vi "computer_GUI.vi"(11 "GUI_cluster":T2={"Sub Panel"=refnum, "GUIdevice"="Bella_LP_Mode", "CtlRef"=refnum, "User Event in"=refnum}) -> ()   [LabVIEW 2013]
uses:
  Shared/GUI_Template/GUI_master/tcp new data cluster.ctl
  Controls/eventtypdef1.ctl
  <vilib>/Utility/miscctls.llb/LVRangeTypeDef.ctl
  Shared/GUI_Template/GUI_master/tcp_new_data_event.ctl
  Controls/GUI_cluster.ctl
panel:
  out "Slide 2":u8(slide) scale=0.0..100.0
  in  "Refresh Button":bool
  in  "check coputers":bool=TRUE
  out "All on?":bool
  out "Computers not on":string[](array[string])
  out "off computers":string[](array[string])
  in  "Ping type":T1(ring)
  in  "IP Addresses":string[](array[string])
  in  "error out":errorcluster
  out "error out 2":errorcluster
  out "tcp data event":T3
  out "GUIdevice 1":string="Bella_LP_Mode"
  in  "stop":bool
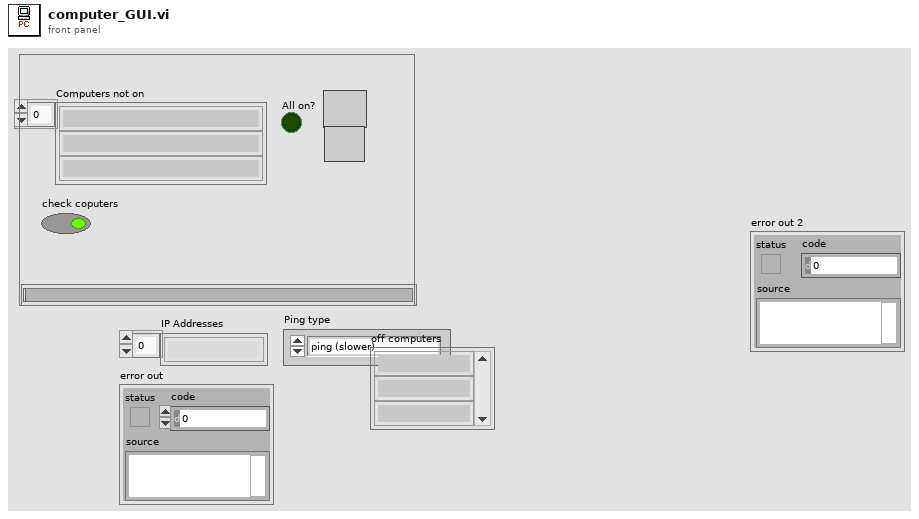
[diagram p1: front panel]
types:
  T1 = enum16{"ping (slower)", "nmap (only if installed)"}
  T2 = typedef "GUI_cluster.ctl" = cluster{"Sub Panel":refnum<vi>, "GUIdevice":string, "CtlRef":refnum<vi>, "User Event in":refnum<user-event>}
  T3 = typedef "tcp_new_data_event.ctl" = refnum<user-event>
  T4 = typedef "eventtypdef1.ctl" = cluster{"label":string, "Sub Panel":refnum<vi>, "CtlRef":refnum<vi>, "This VI":refnum<vi>}
  T5 = typedef "tcp new data cluster.ctl" = cluster{"EventEnum":enum16{"new data", "connection status update"}, "Device name":string}
  T6 = typedef "LVRangeTypeDef.ctl" = cluster{"Minimum":dbl, "Maximum":dbl, "Increment":dbl, "Minor Increment":dbl, "Start":dbl}
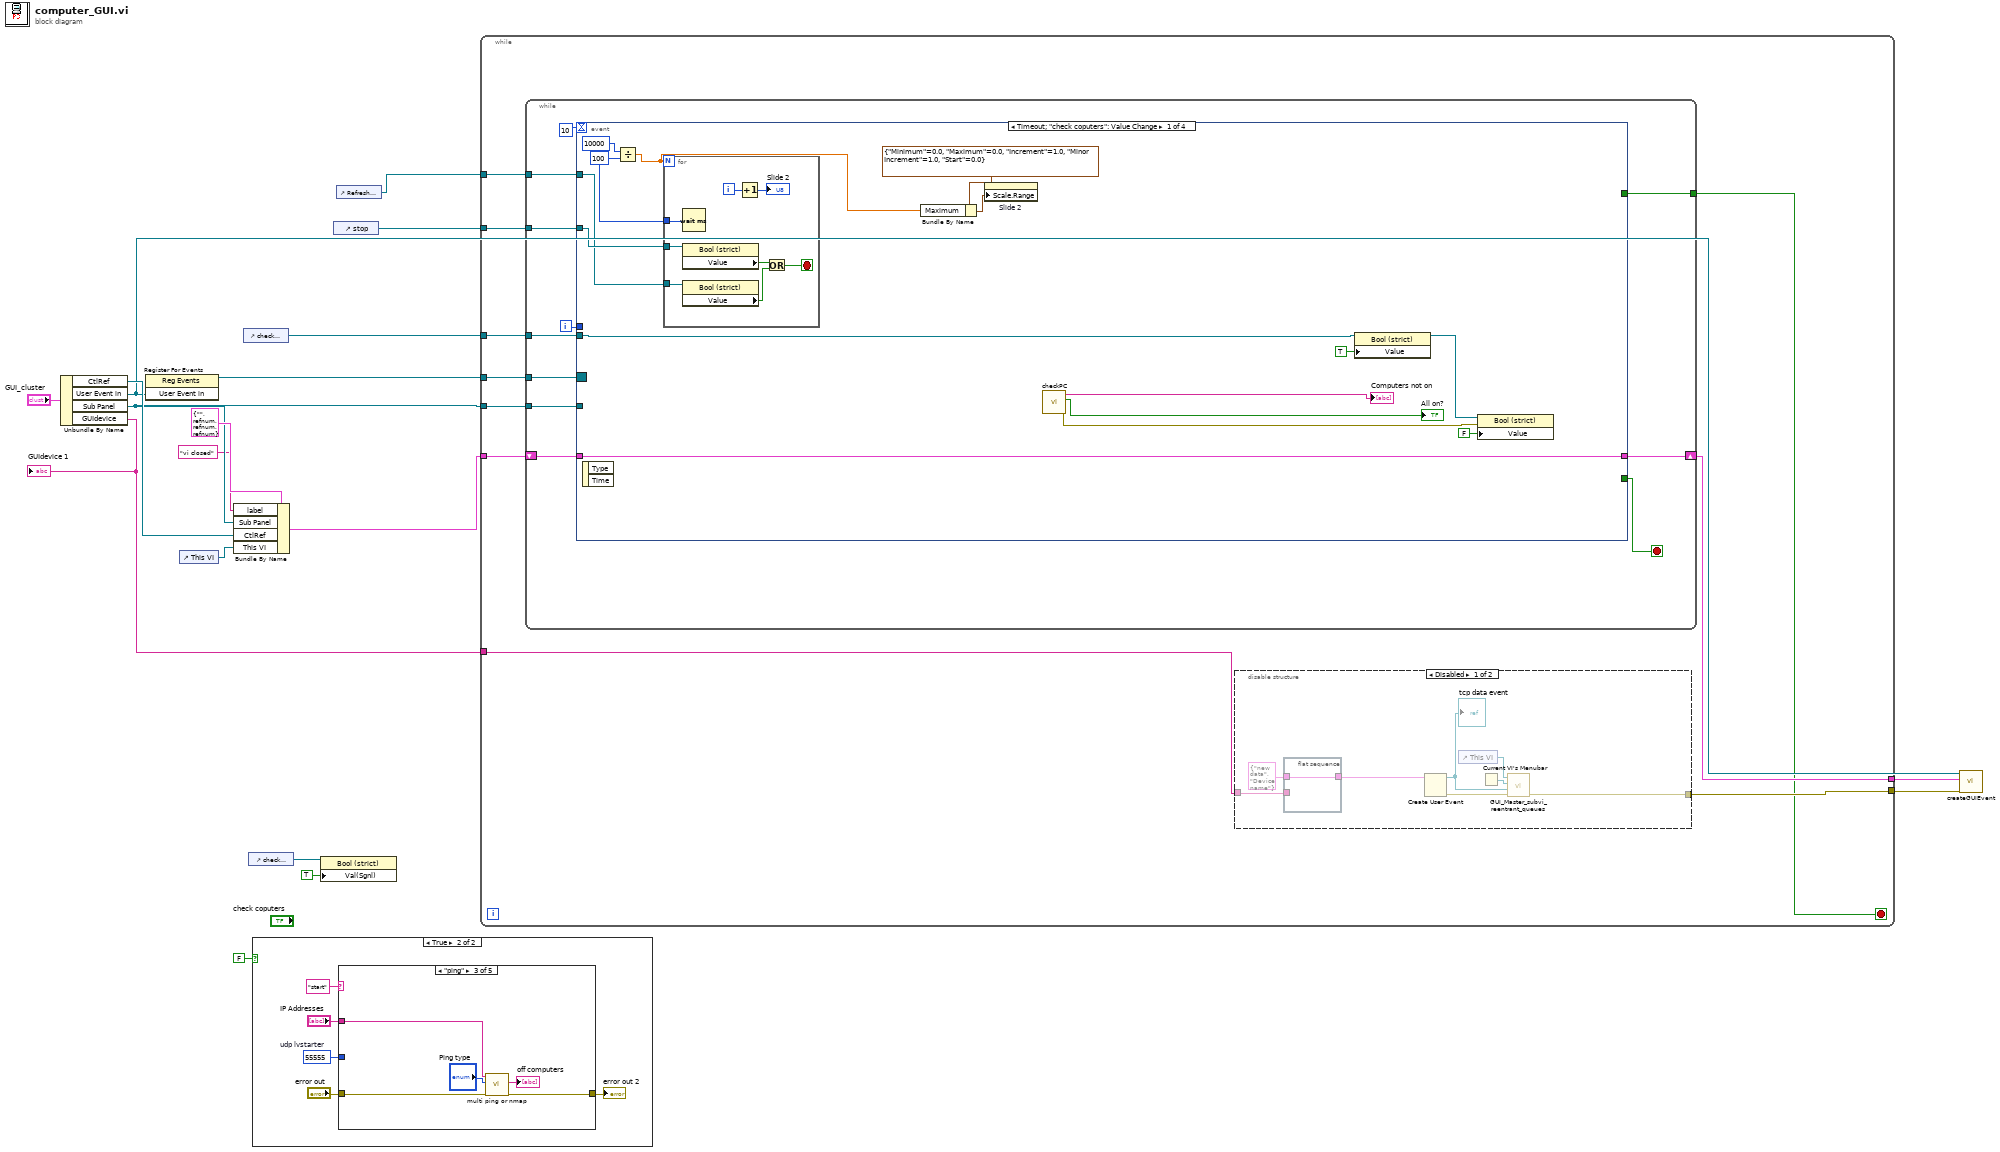
[diagram p0: block diagram]
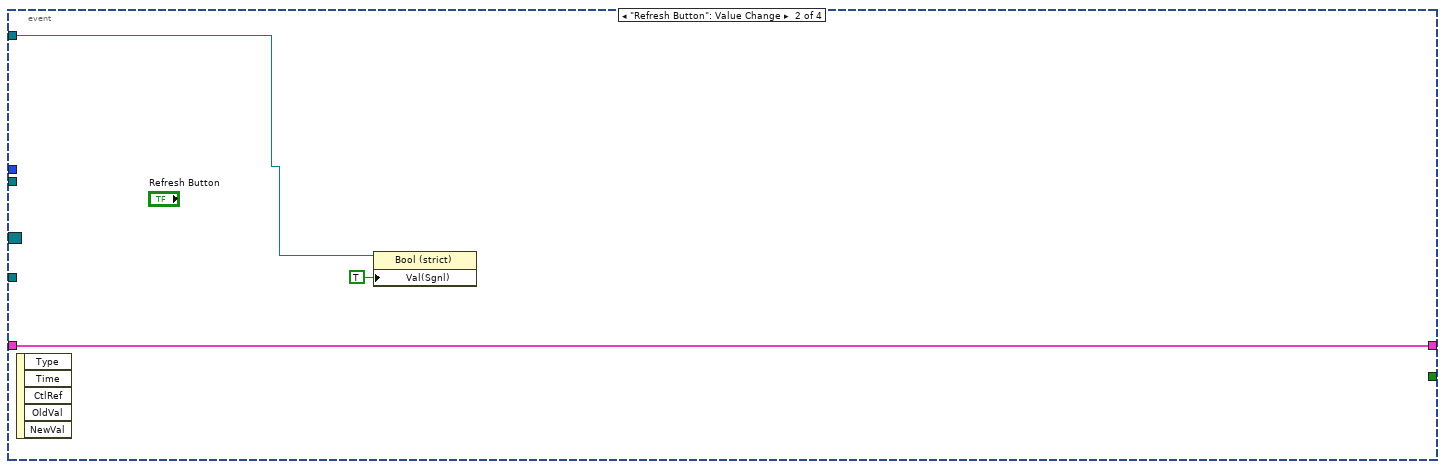
[diagram p3: hidden frame]
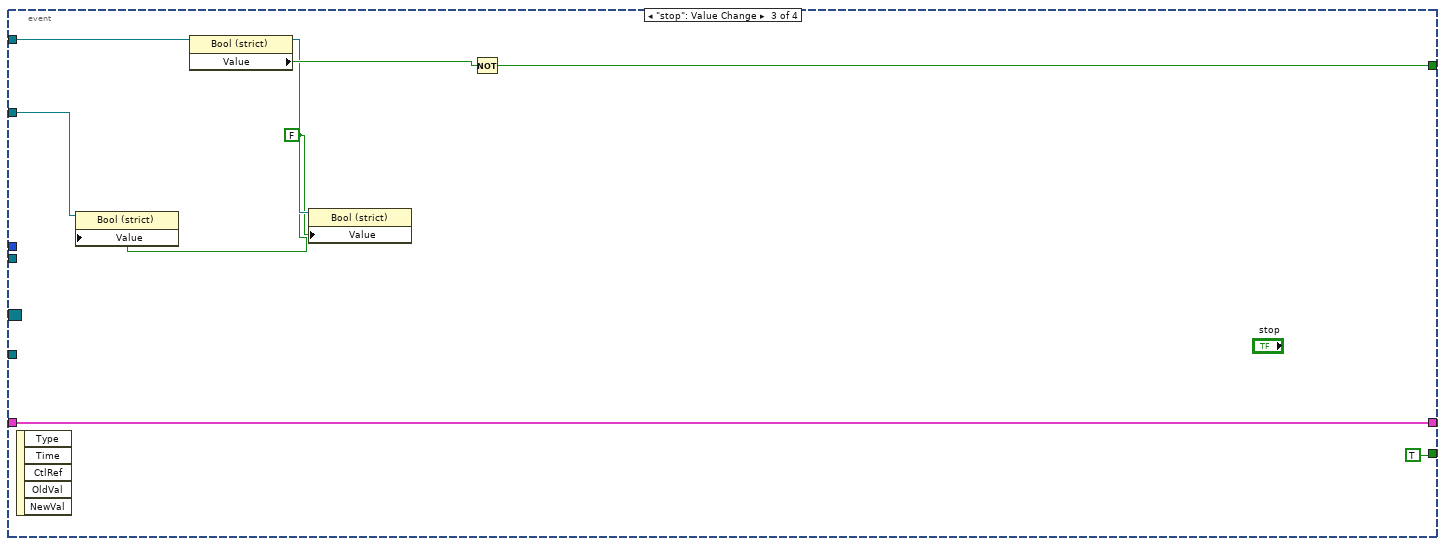
[diagram p4: hidden frame]
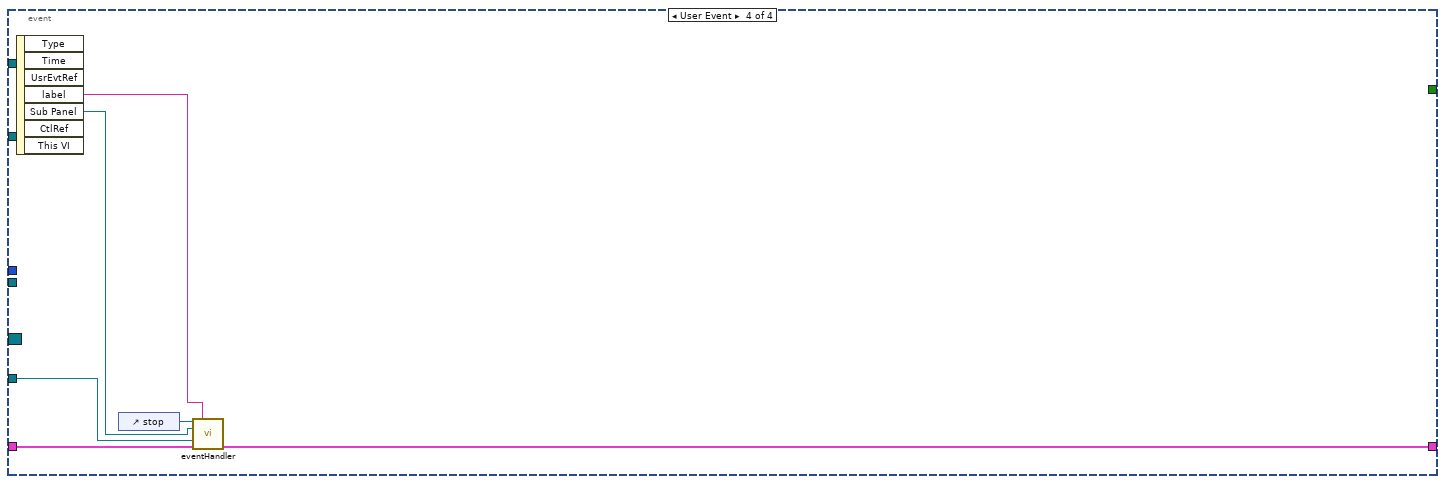
[diagram p5: hidden frame]
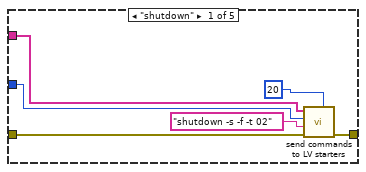
[diagram p7: hidden frame]
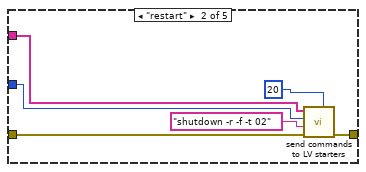
[diagram p8: hidden frame]
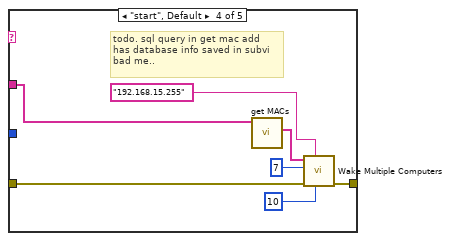
[diagram p9: hidden frame]
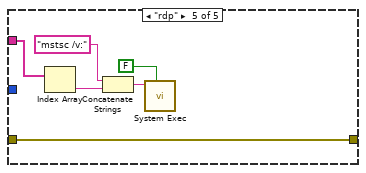
[diagram p10: hidden frame]
diagram:
  n1 = Unbundle By Name("GUI_cluster") -> ("CtlRef"=w16:refnum<vi>, "User Event in"=w11:refnum<user-event>, "Sub Panel"=w9:refnum<vi>, "GUIdevice"=w14:string)
  "GUIdevice 1" <- w14
  n2 = register-events(w11) -> (reference out=w10:refnum<event-registration>)  [unwired: 2 in, 1 out]
  n3 = control-ref of="This VI"() -> (w15:refnum<vi>)
  n4 = Bundle By Name(cluster=T4 {"label"="", "Sub Panel"=refnum, "CtlRef"=refnum, "This VI"=refnum} ("event data"), "label"="vi closed", "Sub Panel"=w9, "CtlRef"=w16, "This VI"=w15) -> (w12:T4)
  n5 = control-ref of="check coputers"() -> (w3:refnum<vi>)
  n6 = control-ref of="check coputers"() -> (w5:refnum<vi>)
  n7 = case shown="True" FALSE {
    frame False {
    }
    frame True {
      w20 = u16 55555  # udp lvstarter
      n8 = case shown="\"ping\"" "start" {
        tunnel: "IP Addresses" -> [w29 w35 w39 w43 w51]
        tunnel: w20 -> [w28 w34 _ _ _]
        tunnel: "error out" -> [w26 w32 w36 w45 w53]
        tunnel: [w25 w31 w38 w44 w53] -> w21
        frame "shutdown" {
          n9 = call "send commands to LV starters.vi"("IP Addresses"=w29, "Local Port"=w28, "Message"="shutdown -s -f -t 02", "error in"=w26, "time between commands (ms)"=u32 20) -> ("error out"=w25:errorcluster)  [unwired: 3 in, 1 out]
        }
        frame "restart" {
          n10 = call "send commands to LV starters.vi"("IP Addresses"=w35, "Local Port"=w34, "Message"="shutdown -r -f -t 02", "error in"=w32, "time between commands (ms)"=u32 20) -> ("error out"=w31:errorcluster)  [unwired: 3 in, 1 out]
        }
        frame "ping" {
          n11 = call "multi ping or nmap.vi"("error in (no error)"=w36, "Ping type"="Ping type", "IP Addresses"=w39) -> ("error out"=w38:errorcluster, "Computers not on"=→"off computers":string[])  [unwired: 2 in, 1 out]
        }
        frame "start", Default {
          # "todo. sql query in get mac add\nhas database info saved in subvi\nbad me.."
          n12 = call "get MACs.vi"("IP Addresses to..."=w43) -> ("MACs Hex"=w42:string[])  [unwired: 9 in, 1 out]
          n13 = call "Wake Multiple Computers.vi"("wait in between [ms]"=u32 10, "Broadcast IP-address"="192.168.15.255", "error in"=w45, "local port"=u16 7, "MAC Addresses to Start"=w42) -> ("error out"=w44:errorcluster)  [unwired: 6 in]
        }
        frame "rdp" {
          n14 = Index Array(array=w51) -> (element=w50:string)  [unwired: 1 in]
          n15 = Concatenate Strings("mstsc /v:" ("IP"), w50) -> (w48:string)
          n16 = call <vilib>:"System Exec.vi"("wait until completion? (T)"=FALSE, "command line"=w48) -> ()  [unwired: 4 in, 6 out]
        }
      }
      "error out 2" <- w21
    }
  }
  n17 = property class="Bool (strict)"(reference=w5, "Val(Sgnl)"=TRUE ("Value (Signaling)")) -> ()  [unwired: 1 in, 2 out]
  n18 = control-ref of="stop"() -> (w2:refnum<vi>)
  n19 = control-ref of="Refresh Button"() -> (w1:refnum<vi>)
  n20 = while {
    tunnel: w14 -> [w63]
    tunnel: [w62] -> w13
    tunnel: w12 -> [w61]
    tunnel: w10 -> [w60]
    tunnel: w9 -> [w59]
    tunnel: [w58] -> w8
    tunnel: w3 -> [w57]
    tunnel: w2 -> [w56]
    tunnel: w1 -> [w55]
    stop <- w54 stop-if-true
    n21 = while {
      shift-right: [w82] -> w58
      shift-left: w61 -> [w83]
      tunnel: w60 -> [w81]
      tunnel: w59 -> [w80]
      tunnel: w57 -> [w77]
      tunnel: w56 -> [w75]
      tunnel: w55 -> [w74]
      tunnel: [w73] -> w54
      i -> [w78]
      stop <- w76 stop-if-true
      n22 = event shown="[0] Timeout;  \"check coputers\": Value Change" {
        selector: w81 -> [_ _ _ _]
        dyn-events: _ -> [_ _ _ _]
        timeout: 10 -> [_ _ _ _]
        tunnel: [_ _ TRUE ("stop") _] -> w76
        tunnel: w83 -> [w98 w107 w117 w120]
        tunnel: [w98 w107 w117 w119] -> w82
        tunnel: w80 -> [_ _ _ w121]
        tunnel: w78 -> [_ _ _ _]
        tunnel: w77 -> [w95 _ _ _]
        tunnel: w75 -> [w85 w108 w111 _]
        tunnel: w74 -> [w84 _ w116 _]
        tunnel: [_ _ w114 _] -> w73
        event Timeout; "check coputers": Value Change {
          w87 = 100 ("y")
          n23 = event-data() -> ()  [unwired: 1 in, 2 out]
          n24 = Divide(x=10000 ("y"), y=w87) -> (x/y=w90:dbl)
          n25 = for {
            N: w90 -> [_]
            tunnel: w87 -> [w104]
            tunnel: w85 -> [w103]
            tunnel: w84 -> [w102]
            i -> [w106]
            stop <- w99 stop-if-true
            n26 = Wait (ms)(milliseconds to wait=w104) -> ()  [unwired: 1 out]
            n27 = property class="Bool (strict)"(reference=w103) -> ("Value"=w101:bool)  [unwired: 1 in, 2 out]
            n28 = property class="Bool (strict)"(reference=w102) -> ("Value"=w100:bool)  [unwired: 1 in, 2 out]
            n29 = Increment(x=w106) -> (x+1=→"Slide 2":i32)
            n30 = Or(x=w101, y=w100) -> (x .or. y?=w99:bool)
          }
          n31 = Bundle By Name(cluster=T6 {"Minimum"=0.0, "Maximum"=0.0, "Increment"=1.0, "Minor Increment"=1.0, "Start"=0.0} ("Scale.Range"), "Maximum"=w90) -> (w88:T6)
          n32 = property on="Slide 2" class="Slide (strict)"("Scale.Range"=w88) -> ()  [unwired: 2 in, 2 out]
          n33 = call "checkPC.vi"() -> ("error out"=w93:errorcluster, "All on?"=→"All on?":bool, "Computers not on"=→"Computers not on":string[])  [unwired: 9 in]
          n34 = property class="Bool (strict)"(reference=w95, "Value"=TRUE ("Value (Signaling)")) -> (reference out=w91:refnum<vi>)  [unwired: 1 in, 1 out]
          n35 = property class="Bool (strict)"(reference=w91, error in=w93, "Value"=FALSE) -> ()  [unwired: 2 out]
        }
        event "Refresh Button": Value Change {
          n36 = event-data() -> ()  [unwired: 1 in, 5 out]
          n37 = property class="Bool (strict)"(reference=w108, "Val(Sgnl)"=TRUE ("Value (Signaling)")) -> ()  [unwired: 1 in, 2 out]
        }
        event "stop": Value Change {
          w110 = FALSE ("Value")
          n38 = event-data() -> ()  [unwired: 1 in, 5 out]
          n39 = property class="Bool (strict)"(reference=w111, "Value"=w110) -> ()  [unwired: 1 in, 2 out]
          n40 = property class="Bool (strict)"(reference=w116) -> (reference out=w112:refnum<vi>, "Value"=w115:bool)  [unwired: 1 in, 1 out]
          n41 = property class="Bool (strict)"(reference=w112, "Value"=w110) -> ()  [unwired: 1 in, 2 out]
          n42 = Not(x=w115) -> (.not. x?=w114:bool)
        }
        event User Event {
          n43 = event-data() -> ("label"=w118:string, "Sub Panel"=w122:refnum<vi>)  [unwired: 1 in, 5 out]
          n44 = control-ref of="stop"() -> (w123:refnum<vi>)
          n45 = call "eventHandler.vi"("Boolean in"=w123, "label"=w118, "Sub Panel 2"=w122, "Sub Panel"=w121, "event data in"=w120) -> ("event data out"=w119:T4)  [unwired: 10 in]
        }
      }
    }
    n46 = disable-structure shown="Disabled" {
      disable-tunnel: w63 -> [w65 _]
      disable-tunnel: [w64 _] -> w62
      frame Disabled {
        n47 = flat-sequence {
          tunnel: T5 {"EventEnum"=enum."new data", "Device name"="Device name"} ("New Event") -> [w72]
          tunnel: [w72] -> w66
          tunnel: w65 -> [_]
          frame #0 {
          }
        }
        n48 = Create User Event(user event datatype=w66) -> (user event=w68:refnum<user-event>, error out=w69:errorcluster)  [unwired: 1 in]
        "tcp data event" <- w68
        n49 = control-ref of="This VI"() -> (w71:refnum<vi>)
        n50 = Current VI's Menubar() -> (w70:refnum<k9>)
        n51 = call "GUI_Master_subvi_reentrant_queues.vi"("error in (no error)"=w69, "tcp data event"=w68, "Caller menu reference"=w70, "Caller VI ref"=w71) -> ("error out"=w64:errorcluster)  [unwired: 7 in]
      }
      frame Enabled {
      }
    }
  }
  n52 = call "createGUIEvent.vi"("error in (no error)"=w13, "event data"=w8, "User Event in"=w11) -> ()  [unwired: 8 in, 1 out]
